vi "APIRestRequest.vi"(7 "API Token":string, 8 "error in (no error)":errorcluster, 9 "Argument":string, 10 "Base URL":string, 11 "API GET":T1(ring)) -> (0 "error out":errorcluster, 2 "body":string, 3 "headers":string)   [LabVIEW 2020, in "StashRoyale.lvclass"]
uses:
  StashRoyale.lvclass
  <vilib>/httpClient/LabVIEWHTTPClient.lvlib
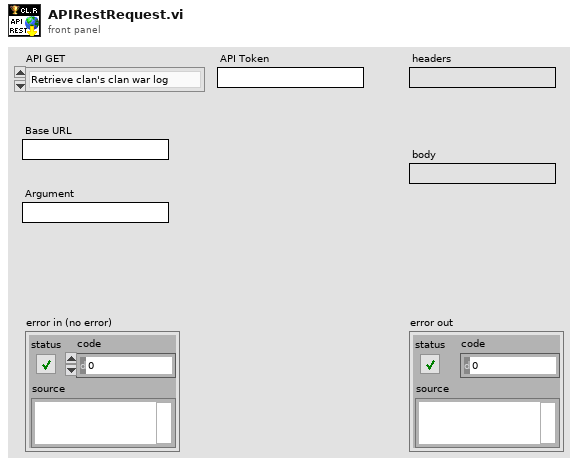
[diagram p1: front panel]
types:
  T1 = enum16{"Retrieve clan's clan war log", "Search clans", "Retrieve clan's river race log", "Retrieve information about clan's current clan war", "Get clan information", "List clan members", "Retrieve information about clan's current river race", "Get player information", "Get information about player's upcoming chests", "Get list of recent battles for a player", "Get list of available cards", "Search tournaments", "Get tournament information", "Get clan rankings for a specific location", "Get player rankings for a specific location", "Get clan war rankings for a specific location", "Get top Path of Legend players for given season", "Get top player league season", "Get top player rankings for a season", "Lists top player league seasons.", "List locations", "Get location information", "Get current and upcoming challenges", "Get list of global tournaments"}
  T2 = typedef "LabVIEWHTTPClient.lvlib/ClientHandle.ctl" = refnum<k1>
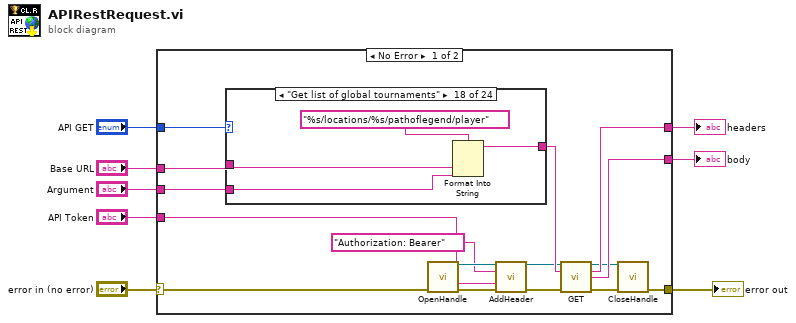
[diagram p0: block diagram]
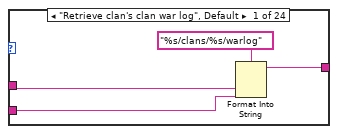
[diagram p2: hidden frame]
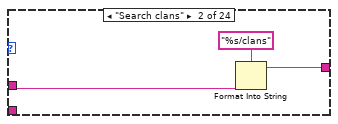
[diagram p3: hidden frame]
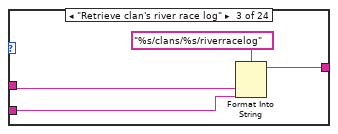
[diagram p4: hidden frame]
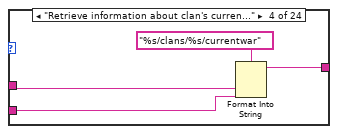
[diagram p5: hidden frame]
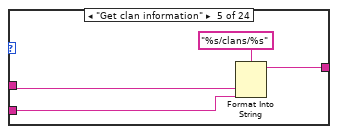
[diagram p6: hidden frame]
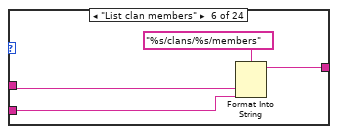
[diagram p7: hidden frame]
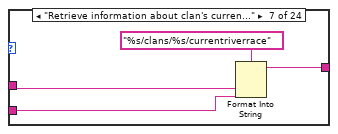
[diagram p8: hidden frame]
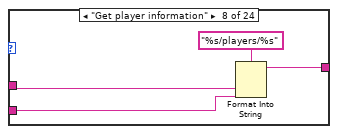
[diagram p9: hidden frame]
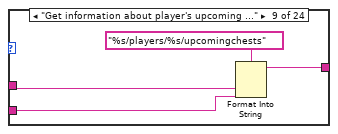
[diagram p10: hidden frame]
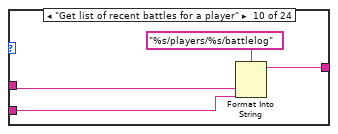
[diagram p11: hidden frame]
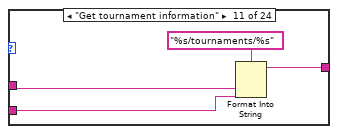
[diagram p12: hidden frame]
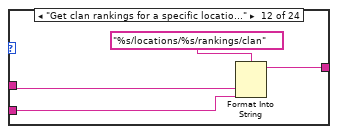
[diagram p13: hidden frame]
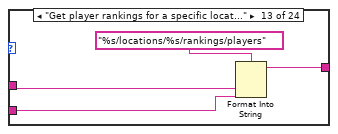
[diagram p14: hidden frame]
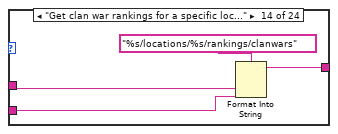
[diagram p15: hidden frame]
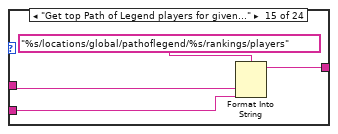
[diagram p16: hidden frame]
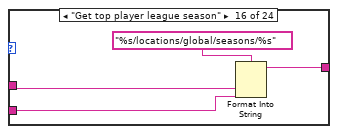
[diagram p17: hidden frame]
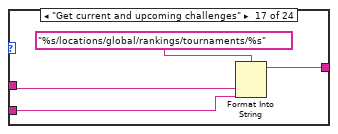
[diagram p18: hidden frame]
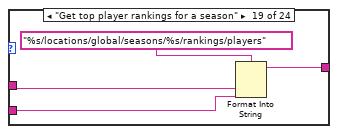
[diagram p19: hidden frame]
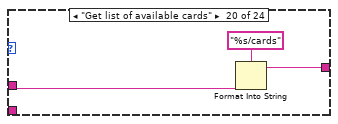
[diagram p20: hidden frame]
diagram:
  n1 = case shown="No Error" "error in (no error)" {
    selector: "error in (no error)" -> [w12 w116]
    tunnel: "Argument" -> [w24 _]
    tunnel: "API GET" -> [w23 _]
    tunnel: "Base URL" -> [w21 _]
    tunnel: [w20 _] -> w5
    tunnel: "API Token" -> [w19 _]
    tunnel: [w13 w116] -> w3
    tunnel: [w11 _] -> w1
    frame No Error {
      n2 = case shown="\"Get list of global tournaments\"" w23 {
        tunnel: w21 -> [w28 w31 w35 w39 w43 w47 w51 w55 w59 w63 w67 w71 w75 w79 w83 w87 w91 w95 w99 w102 w105 w108 w112 w115]
        tunnel: [w26 w29 w33 w37 w41 w45 w49 w53 w57 w61 w65 w69 w73 w77 w81 w85 w89 w93 w97 w100 w103 w106 w110 w113] -> w22
        tunnel: w24 -> [w25 _ w32 w36 w40 w44 w48 w52 w56 w60 w64 w68 w72 w76 w80 w84 w88 w92 w96 _ _ _ w109 _]
        frame "Retrieve clan's clan war log", Default {
          n3 = Format Into String(format string="%s/clans/%s/warlog" ("url"), w28, w25) -> (resulting string=w26:string)  [unwired: 2 in, 1 out]
        }
        frame "Search clans" {
          n4 = Format Into String(format string="%s/clans" ("url"), w31) -> (resulting string=w29:string)  [unwired: 2 in, 1 out]
        }
        frame "Retrieve clan's river race log" {
          n5 = Format Into String(format string="%s/clans/%s/riverracelog" ("url"), w35, w32) -> (resulting string=w33:string)  [unwired: 2 in, 1 out]
        }
        frame "Retrieve information about clan's current clan war" {
          n6 = Format Into String(format string="%s/clans/%s/currentwar" ("url"), w39, w36) -> (resulting string=w37:string)  [unwired: 2 in, 1 out]
        }
        frame "Get clan information" {
          n7 = Format Into String(format string="%s/clans/%s" ("url"), w43, w40) -> (resulting string=w41:string)  [unwired: 2 in, 1 out]
        }
        frame "List clan members" {
          n8 = Format Into String(format string="%s/clans/%s/members" ("url"), w47, w44) -> (resulting string=w45:string)  [unwired: 2 in, 1 out]
        }
        frame "Retrieve information about clan's current river race" {
          n9 = Format Into String(format string="%s/clans/%s/currentriverrace" ("url"), w51, w48) -> (resulting string=w49:string)  [unwired: 2 in, 1 out]
        }
        frame "Get player information" {
          n10 = Format Into String(format string="%s/players/%s" ("url"), w55, w52) -> (resulting string=w53:string)  [unwired: 2 in, 1 out]
        }
        frame "Get information about player's upcoming chests" {
          n11 = Format Into String(format string="%s/players/%s/upcomingchests" ("url"), w59, w56) -> (resulting string=w57:string)  [unwired: 2 in, 1 out]
        }
        frame "Get list of recent battles for a player" {
          n12 = Format Into String(format string="%s/players/%s/battlelog" ("url"), w63, w60) -> (resulting string=w61:string)  [unwired: 2 in, 1 out]
        }
        frame "Get tournament information" {
          n13 = Format Into String(format string="%s/tournaments/%s" ("url"), w67, w64) -> (resulting string=w65:string)  [unwired: 2 in, 1 out]
        }
        frame "Get clan rankings for a specific location" {
          n14 = Format Into String(format string="%s/locations/%s/rankings/clan" ("url"), w71, w68) -> (resulting string=w69:string)  [unwired: 2 in, 1 out]
        }
        frame "Get player rankings for a specific location" {
          n15 = Format Into String(format string="%s/locations/%s/rankings/players" ("url"), w75, w72) -> (resulting string=w73:string)  [unwired: 2 in, 1 out]
        }
        frame "Get clan war rankings for a specific location" {
          n16 = Format Into String(format string="%s/locations/%s/rankings/clanwars" ("url"), w79, w76) -> (resulting string=w77:string)  [unwired: 2 in, 1 out]
        }
        frame "Get top Path of Legend players for given season" {
          n17 = Format Into String(format string="%s/locations/global/pathoflegend/%s/rankings/players" ("url"), w83, w80) -> (resulting string=w81:string)  [unwired: 2 in, 1 out]
        }
        frame "Get top player league season" {
          n18 = Format Into String(format string="%s/locations/global/seasons/%s" ("url"), w87, w84) -> (resulting string=w85:string)  [unwired: 2 in, 1 out]
        }
        frame "Get current and upcoming challenges" {
          n19 = Format Into String(format string="%s/locations/global/rankings/tournaments/%s" ("url"), w91, w88) -> (resulting string=w89:string)  [unwired: 2 in, 1 out]
        }
        frame "Get list of global tournaments" {
          n20 = Format Into String(format string="%s/locations/%s/pathoflegend/player" ("url"), w95, w92) -> (resulting string=w93:string)  [unwired: 2 in, 1 out]
        }
        frame "Get top player rankings for a season" {
          n21 = Format Into String(format string="%s/locations/global/seasons/%s/rankings/players" ("url"), w99, w96) -> (resulting string=w97:string)  [unwired: 2 in, 1 out]
        }
        frame "Get list of available cards" {
          n22 = Format Into String(format string="%s/cards" ("url"), w102) -> (resulting string=w100:string)  [unwired: 2 in, 1 out]
        }
        frame "Search tournaments" {
          n23 = Format Into String(format string="%s/tournaments" ("url"), w105) -> (resulting string=w103:string)  [unwired: 2 in, 1 out]
        }
        frame "Lists top player league seasons." {
          n24 = Format Into String(format string="%s/locations/global/seasons" ("url"), w108) -> (resulting string=w106:string)  [unwired: 2 in, 1 out]
        }
        frame "Get location information" {
          n25 = Format Into String(format string="%s/locations/%s" ("url"), w112, w109) -> (resulting string=w110:string)  [unwired: 2 in, 1 out]
        }
        frame "List locations" {
          n26 = Format Into String(format string="%s/locations" ("url"), w115) -> (resulting string=w113:string)  [unwired: 2 in, 1 out]
        }
      }
      n27 = call <vilib>:"OpenHandle.vi"("error in (no error)"=w12) -> ("client handle out"=w15:T2, "error out"=w18:errorcluster)  [unwired: 13 in]
      n28 = call <vilib>:"AddHeader.vi"("client handle"=w15, "header"="Authorization: Bearer", "value"=w19, "error in (no error)"=w18) -> ("client handle out"=w16:T2, "error out"=w17:errorcluster)  [unwired: 10 in]
      n29 = call <vilib>:"GET.vi"("client handle"=w16, "url"=w22, "error in (no error)"=w17) -> ("client handle out"=w9:T2, "headers"=w20:string, "body"=w11:string, "error out"=w10:errorcluster)  [unwired: 9 in]
      n30 = call <vilib>:"CloseHandle.vi"("client handle"=w9, "error in (no error)"=w10) -> ("error out"=w13:errorcluster)  [unwired: 13 in]
    }
    frame Error {
    }
  }
  "headers" <- w5
  "error out" <- w3
  "body" <- w1
